vi "Initialize Console Options.vi"(8 "error in (no error)":errorcluster, 11 "Entry Console View Definition in":refnum<class "Entry Console View Definition.lvclass">) -> (0 "error out":errorcluster, 3 "Entry Console View Definition out":refnum<class "Entry Console View Definition.lvclass">)   [LabVIEW 2019, in "Entry Console View Definition.lvclass"]
uses:
  <vilib>/gpm_packages/@cs/Car-wash/Source/Entry Console View Definition/Entry Console View Definition/Entry Console View Definition.lvclass
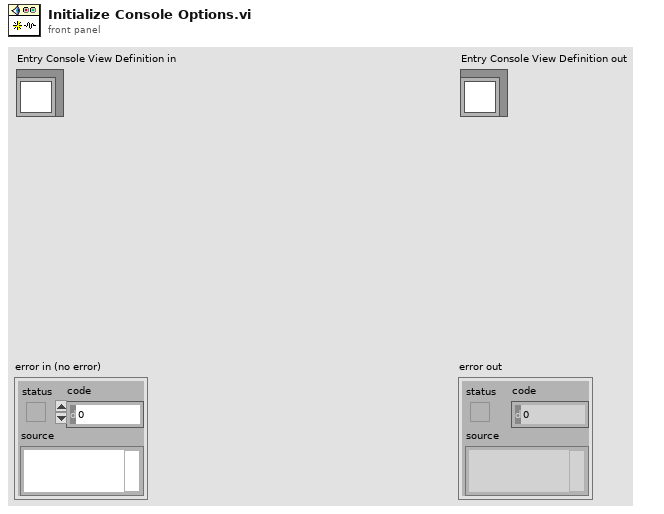
[diagram p1: front panel]
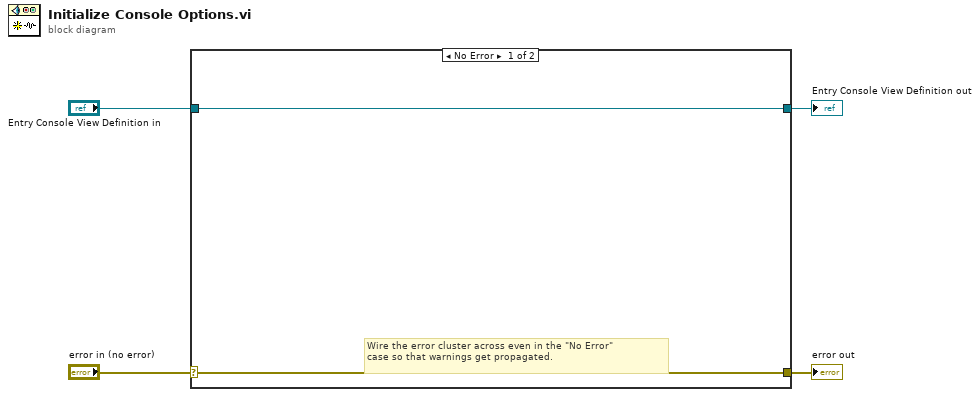
[diagram p0: block diagram]
diagram:
  n1 = case shown="No Error" "error in (no error)" {
    selector: "error in (no error)" -> [w5 w8]
    tunnel: [w5 w8] -> w3
    tunnel: [w6 w7] -> w1
    tunnel: "Entry Console View Definition in" -> [w6 w7]
    frame No Error {
      # "Wire the error cluster across even in the \"No Error\"\ncase so that warnings get propagated."
    }
    frame Error {
    }
  }
  "error out" <- w3
  "Entry Console View Definition out" <- w1
